vi "WSVCAP SHL Host LL I2C Read.vi"(0 "Bytes to Read":u8=8, 1 "Wait Ticks":u32, 2 "Slave Address":u8, 5 "Sub Address [U8]":u8=191 format="%.0x", 7 "Socket Mask [U64]":u64=1 format="%06x", 11 "error in":errorcluster, 12 "UUT Set (0/1)":u8, 13 "FPGA":T1) -> (4 "Cap1:24 Read Data":u8[][](array[numeric]), 14 "Status":u8[](array[numeric]) format="%.0x", 15 "error out":errorcluster)   [LabVIEW 2017]
uses:
  Type Defs/WSVCAP SHL FPGA Enum.ctl
  Type Defs/WSVCAP SHL Top Level Write Read State Enum.ctl
  Type Defs/WSVCAP SHL State.ctl
  Type Defs/WSVCAP SHL Transaction Enum.ctl
  Type Defs/WSVCAP SHL Top Level Control Enum.ctl
  WSVCAP SHL Host LL I2C Debug Global.vi
panel:
  out "Bit Array":u64[](array[numeric]) format="%.0x"
  out "Data Headers":u8[](array[numeric])=[1, 2, 3, 4, 5, 6, 7, 8, 9, 10, 11, 12, 12, 14, 15, 16]
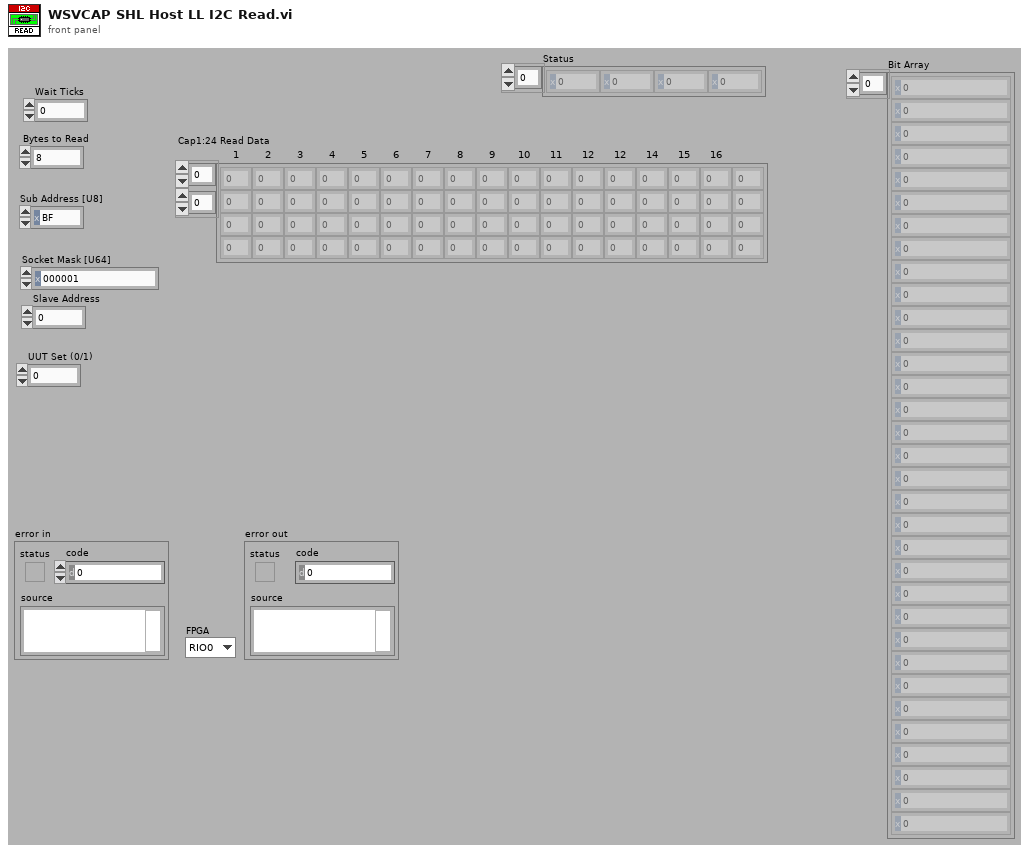
[diagram p1: front panel]
types:
  T1 = typedef "WSVCAP SHL FPGA Enum.ctl" = enum16{"RIO0", "RIO1"}
  T2 = typedef "WSVCAP SHL Top Level Write Read State Enum.ctl" = enum16{"Start", "Write", "Read", "Get Status", "Wait Until Done"}
  T3 = typedef "WSVCAP SHL Transaction Enum.ctl" = enum16{"I2C-Read Data", "I2C-Write Data", "RFFE-Ext Write", "RFFE-Ext Read", "SRL-Write Data"}
  T4 = typedef "WSVCAP SHL Top Level Control Enum.ctl" = enum16{"Start", "Cmd", "Transaction", "Wait Ticks", "Socket Mask", "UUT Set", "Slave Address", "Sub Address", "Bytes to Write", "Bytes to Read", "Write Data", "Write Flag", "Read Data", "Read Flag", "Ack Read", "Read Status Flag", "Ack Read Status", "Status", "Cycle Count", "Stop Cycle", "Exit"}
  T5 = typedef "WSVCAP SHL State.ctl" = enum8{"Idle", "Transfer Data"}
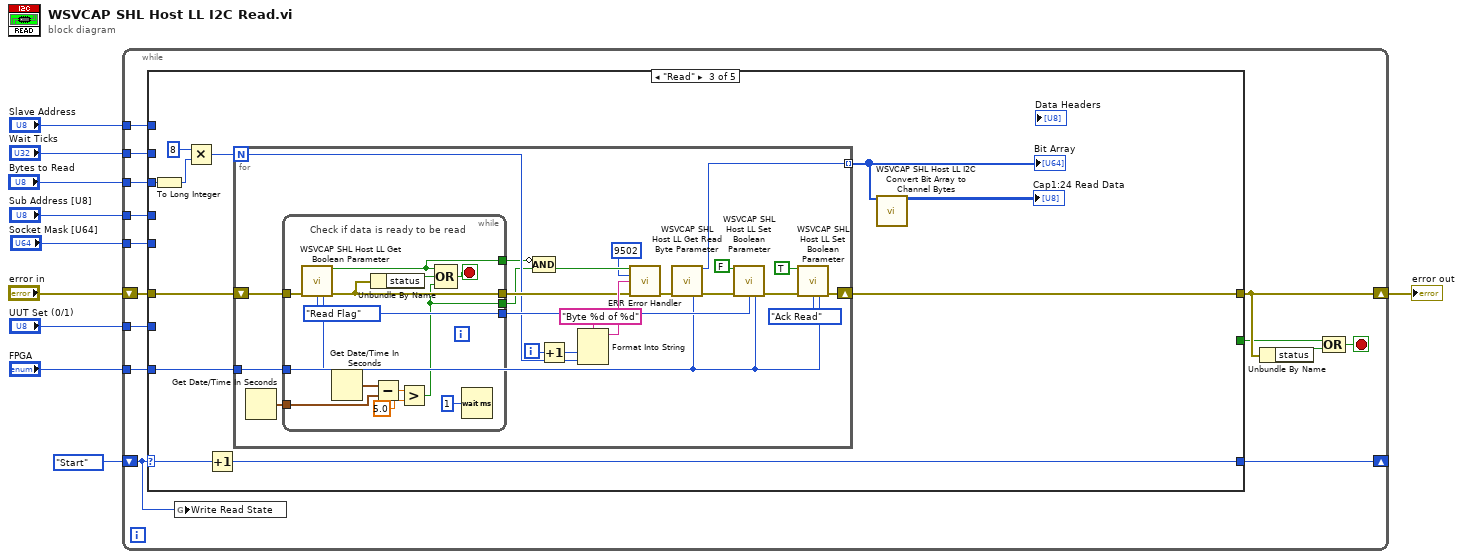
[diagram p0: block diagram]
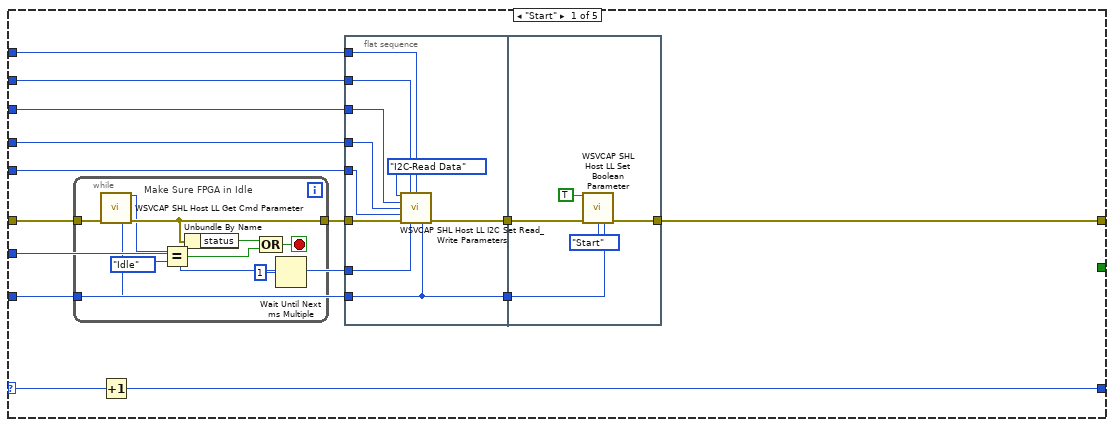
[diagram p2: hidden frame]
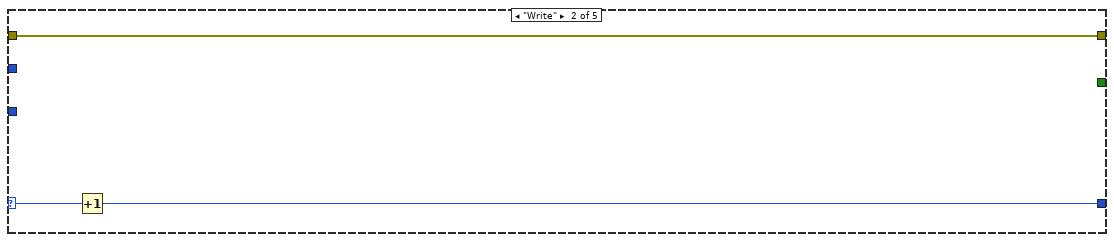
[diagram p3: hidden frame]
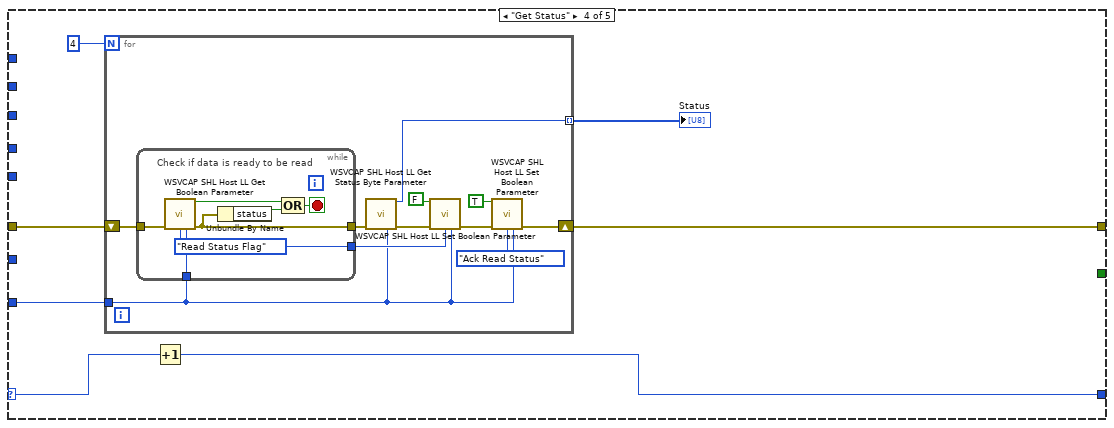
[diagram p4: hidden frame]
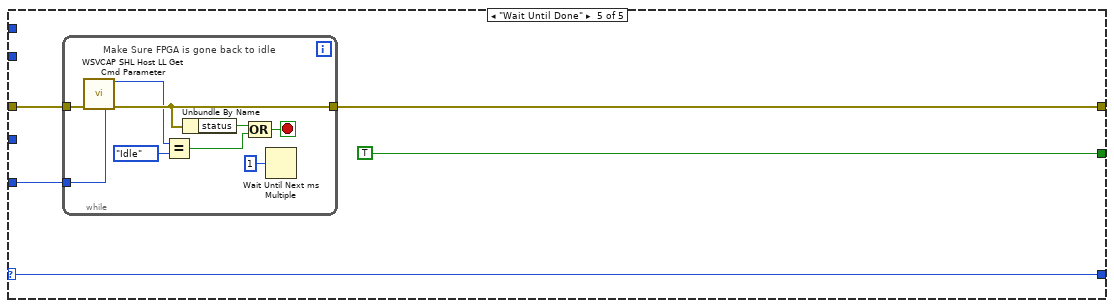
[diagram p5: hidden frame]
diagram:
  n1 = while {
    shift-right: [w23] -> w9
    shift-left: "error in" -> [w24]
    shift-right: [w19] -> _
    shift-left: WSVCAP_SHL_Top_Level_Write_Read_State_Enum."Start" ("Write Read State") -> [w11]
    tunnel: "Bytes to Read" -> [w18]
    tunnel: "Sub Address [U8]" -> [w17]
    tunnel: "Socket Mask [U64]" -> [w16]
    tunnel: "Wait Ticks" -> [w15]
    tunnel: "Slave Address" -> [w14]
    tunnel: "UUT Set (0/1)" -> [w13]
    tunnel: "FPGA" -> [w12]
    stop <- w20 stop-if-true
    n2 = case shown="\"Read\"" w11 {
      selector: w11 -> [w37 w63 w74 w115 w138]
      tunnel: w24 -> [w38 w62 w67 w117 w140]
      tunnel: [w33 w62 w75 w116 w139] -> w23
      tunnel: [_ _ _ _ TRUE] -> w22
      tunnel: [w36 w64 w73 w114 w138] -> w19
      tunnel: w18 -> [w35 _ w72 _ _]
      tunnel: w17 -> [w31 _ _ _ _]
      tunnel: w16 -> [w30 _ _ _ _]
      tunnel: w15 -> [w29 _ _ _ _]
      tunnel: w14 -> [w28 _ _ _ _]
      tunnel: w13 -> [w27 _ _ _ _]
      tunnel: w12 -> [w26 _ w65 w111 w136]
      frame "Start" {
        n3 = while {
          tunnel: w38 -> [w57]
          tunnel: [w56] -> w34
          tunnel: w26 -> [w53]
          stop <- w61 stop-if-true
          # "Make Sure FPGA in Idle"
          n4 = call "WSVCAP SHL Host LL Get Cmd Parameter.vi"("error in (no error)"=w57, "FPGA"=w53) -> ("I2C_Cmd"=w55:T5, "error out"=w56:errorcluster)  [unwired: 12 in]
          n5 = Equal?(x=w55, y=WSVCAP_SHL_State."Idle" ("Type")) -> (x = y?=w59:bool)
          n6 = Unbundle By Name(w56) -> ("status"=w54:bool)
          n7 = Compound Arithmetic op=OR(w54, w59) -> (w61:bool)
          n8 = Wait Until Next ms Multiple(millisecond multiple=u32 1) -> ()  [unwired: 1 out]
        }
        n9 = Increment(x=w37) -> (x+1=w36:T2)
        n10 = flat-sequence {
          tunnel: w35 -> [w45]
          tunnel: w34 -> [w48]
          tunnel: [w46] -> w32
          tunnel: w31 -> [w43]
          tunnel: w30 -> [w44]
          tunnel: w29 -> [w42]
          tunnel: w28 -> [w41]
          tunnel: w27 -> [w40]
          tunnel: w26 -> [w39]
          tunnel: [w39] -> w25
          tunnel: [w52] -> w33
          tunnel: w32 -> [w52]
          tunnel: w25 -> [w49]
          frame #0 {
            n11 = call "WSVCAP SHL Host LL I2C Set Read_Write Parameters.vi"("Transaction"=WSVCAP_SHL_Transaction_Enum."I2C-Read Data", "Wait Ticks"=w42, "Slave Address"=w41, "Bytes"=w45, "Sub Address [U8]"=w43, "Socket Mask [U64]"=w44, "error in (no error)"=w48, "UUT Set (0/1)"=w40, "FPGA"=w39) -> ("error out"=w46:errorcluster)  [unwired: 6 in]
          }
          frame #1 {
            n12 = call "WSVCAP SHL Host LL Set Boolean Parameter.vi"("Boolean In"=TRUE, "error in (no error)"=w52, "FPGA Top Level Control"=WSVCAP_SHL_Top_Level_Control_Enum."Start", "FPGA"=w49) -> ()  [unwired: 11 in, 1 out]
          }
        }
      }
      frame "Write" {
        n13 = Increment(x=w63) -> (x+1=w64:T2)
      }
      frame "Read" {
        n14 = To Long Integer(number=w72) -> (32bit integer=w71:i32)
        n15 = Multiply(x=8, y=w71) -> (x*y=w69:i32)
        n16 = Increment(x=w74) -> (x+1=w73:T2)
        n17 = for {
          N: w69 -> [w80]
          shift-right: [w95] -> w75
          shift-left: w67 -> [w97]
          tunnel: [w89] -> w70 mode=indexing
          tunnel: w65 -> [w76]
          i -> [w81]
          n18 = Get Date/Time In Seconds() -> (seconds since 1Jan1904=w77:timestamp)
          n19 = while {
            tunnel: w97 -> [w109]
            tunnel: [w108] -> w83
            tunnel: [w106] -> w94
            tunnel: w77 -> [w103]
            tunnel: [w100] -> w79
            tunnel: [w99] -> w78
            tunnel: w76 -> [w98]
            stop <- w110 stop-if-true
            w106 = WSVCAP_SHL_Top_Level_Control_Enum."Read Flag" ("FPGA Top Level Control")
            # "Check if data is ready to be read"
            n20 = call "WSVCAP SHL Host LL Get Boolean Parameter.vi"("error in (no error)"=w109, "FPGA Top Level Control"=w106, "FPGA"=w98) -> ("Boolean Out"=w100:bool, "error out"=w108:errorcluster)  [unwired: 11 in]
            n21 = Get Date/Time In Seconds() -> (seconds since 1Jan1904=w104:timestamp)
            n22 = Unbundle By Name(w108) -> ("status"=w107:bool)
            n23 = Subtract(x=w104, y=w103) -> (x-y=w102:dbl)
            n24 = Greater?(x=w102, y=5.0) -> (0:w99:bool)
            n25 = Compound Arithmetic op=OR(w100, w107, w99) -> (w110:bool)
            n26 = Wait (ms)(milliseconds to wait=u32 1) -> ()  [unwired: 1 out]
          }
          n27 = Compound Arithmetic op=AND(invert w79, w78) -> (w88:bool)
          n28 = Increment(x=w81) -> (x+1=w84:i32)
          n29 = Format Into String(format string="Byte %d of %d", w84, w80) -> (resulting string=w86:string)  [unwired: 2 in, 1 out]
          n30 = call "ERR Error Handler.vi"("Error Status"=w88, "Error Code"=9502, "Cause Of Error"=w86, "Error In (no error)"=w83) -> ("Error Out"=w82:errorcluster)  [unwired: 11 in]
          n31 = call "WSVCAP SHL Host LL Get Read Byte Parameter.vi"("error in (no error)"=w82, "FPGA"=w76) -> ("Read Data In"=w89:u64, "error out"=w96:errorcluster)  [unwired: 12 in]
          n32 = call "WSVCAP SHL Host LL Set Boolean Parameter.vi"("Boolean In"=FALSE ("Read Flag"), "error in (no error)"=w96, "FPGA Top Level Control"=w94, "FPGA"=w76) -> ("error out"=w90:errorcluster)  [unwired: 11 in]
          n33 = call "WSVCAP SHL Host LL Set Boolean Parameter.vi"("Boolean In"=TRUE ("Write Flag"), "error in (no error)"=w90, "FPGA Top Level Control"=WSVCAP_SHL_Top_Level_Control_Enum."Ack Read", "FPGA"=w76) -> ("error out"=w95:errorcluster)  [unwired: 11 in]
        }
        "Bit Array" <- w70
        n34 = call "WSVCAP SHL Host LL I2C Convert Bit Array to Channel Bytes.vi"("Bit Array"=w70) -> ("Read Data"=→"Cap1:24 Read Data":u8[][])  [unwired: 14 in]
      }
      frame "Get Status" {
        n35 = for {
          N: 4 -> [_]
          shift-right: [w125] -> w116
          shift-left: w117 -> [w128]
          tunnel: [w119] -> w113 mode=indexing
          tunnel: w111 -> [w118]
          n36 = while {
            tunnel: w128 -> [w133]
            tunnel: [w132] -> w127
            tunnel: [w130] -> w124
            tunnel: w118 -> [w129]
            stop <- w135 stop-if-true
            w130 = WSVCAP_SHL_Top_Level_Control_Enum."Read Status Flag" ("FPGA Top Level Control")
            # "Check if data is ready to be read"
            n37 = call "WSVCAP SHL Host LL Get Boolean Parameter.vi"("error in (no error)"=w133, "FPGA Top Level Control"=w130, "FPGA"=w129) -> ("Boolean Out"=w134:bool, "error out"=w132:errorcluster)  [unwired: 11 in]
            n38 = Unbundle By Name(w132) -> ("status"=w131:bool)
            n39 = Compound Arithmetic op=OR(w134, w131) -> (w135:bool)
          }
          n40 = call "WSVCAP SHL Host LL Get Status Byte Parameter.vi"("error in (no error)"=w127, "FPGA"=w118) -> ("I2C Status Byte"=w119:u8, "error out"=w126:errorcluster)  [unwired: 12 in]
          n41 = call "WSVCAP SHL Host LL Set Boolean Parameter.vi"("Boolean In"=FALSE ("Read Flag"), "error in (no error)"=w126, "FPGA Top Level Control"=w124, "FPGA"=w118) -> ("error out"=w120:errorcluster)  [unwired: 11 in]
          n42 = call "WSVCAP SHL Host LL Set Boolean Parameter.vi"("Boolean In"=TRUE ("Write Flag"), "error in (no error)"=w120, "FPGA Top Level Control"=WSVCAP_SHL_Top_Level_Control_Enum."Ack Read Status", "FPGA"=w118) -> ("error out"=w125:errorcluster)  [unwired: 11 in]
        }
        "Status" <- w113
        n43 = Increment(x=w115) -> (x+1=w114:T2)
      }
      frame "Wait Until Done" {
        n44 = while {
          tunnel: w140 -> [w144]
          tunnel: [w143] -> w139
          tunnel: w136 -> [w141]
          stop <- w146 stop-if-true
          # "Make Sure FPGA is gone back to idle"
          n45 = call "WSVCAP SHL Host LL Get Cmd Parameter.vi"("error in (no error)"=w144, "FPGA"=w141) -> ("I2C_Cmd"=w142:T5, "error out"=w143:errorcluster)  [unwired: 12 in]
          n46 = Equal?(x=w142, y=WSVCAP_SHL_State."Idle") -> (x = y?=w147:bool)
          n47 = Unbundle By Name(w143) -> ("status"=w148:bool)
          n48 = Compound Arithmetic op=OR(w148, w147) -> (w146:bool)
          n49 = Wait Until Next ms Multiple(millisecond multiple=u32 1) -> ()  [unwired: 1 out]
        }
      }
    }
    n50 = global write "WSVCAP SHL Host LL I2C Debug Global.vi" "Write Read State"(w11) -> ()
    n51 = Unbundle By Name(w23) -> ("status"=w21:bool)
    n52 = Compound Arithmetic op=OR(w22, w21) -> (w20:bool)
  }
  "error out" <- w9
